vi "log file name.vi"() -> (8 "file name":string)   [LabVIEW 2012]
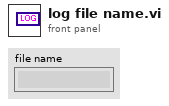
[diagram p1: front panel]
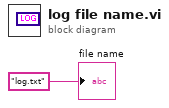
[diagram p0: block diagram]
diagram:
  "file name" <- "log.txt" ("file name")
